vi "getSailingPoints.vi"(10 "sailing points left":i32, 11 "Waypoints":refnum<queue>) -> (2 "remaining sailing points?":bool, 3 "Array":refnum<class "Waypoint.lvclass">[](array[class]))   [LabVIEW 2013]
doc: "Extract remaining sailing points. If none left, returns an empty array."
uses:
  Classes/Waypoint/Waypoint.lvclass
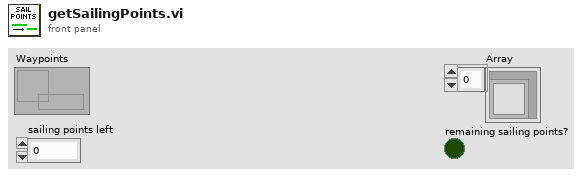
[diagram p1: front panel]
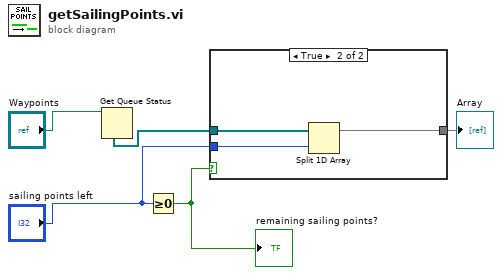
[diagram p0: block diagram]
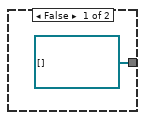
[diagram p2: hidden frame]
diagram:
  n1 = Get Queue Status(queue="Waypoints") -> (elements=w4:refnum<class "Waypoint.lvclass">[])  [unwired: 2 in, 7 out]
  n2 = Greater Or Equal To 0?(x="sailing points left") -> (x >= 0?=w3:bool)
  "remaining sailing points?" <- w3
  n3 = case shown="True" w3 {
    tunnel: w4 -> [_ w9]
    tunnel: "sailing points left" -> [_ w8]
    tunnel: [refnum<class "Waypoint.lvclass">[] [] w7] -> w1
    frame False {
    }
    frame True {
      n4 = Split 1D Array(array=w9, index=w8) -> (first subarray=w7:refnum<class "Waypoint.lvclass">[])  [unwired: 1 out]
    }
  }
  "Array" <- w1
